vi "CoboltLaser_DriveCurrentGet.vi"(0 "ComPort":refnum<visa-resource-name>, 3 "CheckResponse":bool=TRUE, 7 "ErrorIn":errorcluster) -> (20 "ComPortOut":refnum<visa-resource-name>, 21 "LaserCurrent":dbl format="%.3g", 27 "ErrorOut":errorcluster)   [LabVIEW 2019]
doc: "Use this template to build a VI to use as a subVI."
panel:
  out "ResponseOK":bool
  out "Response":string
  # "(mA)"
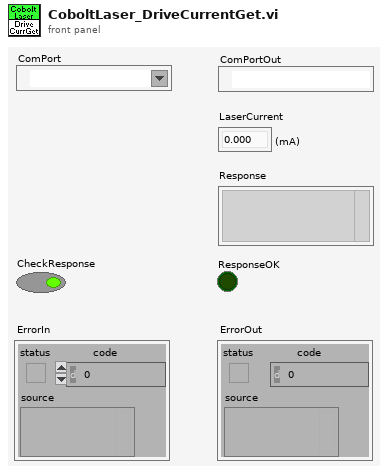
[diagram p1: front panel]
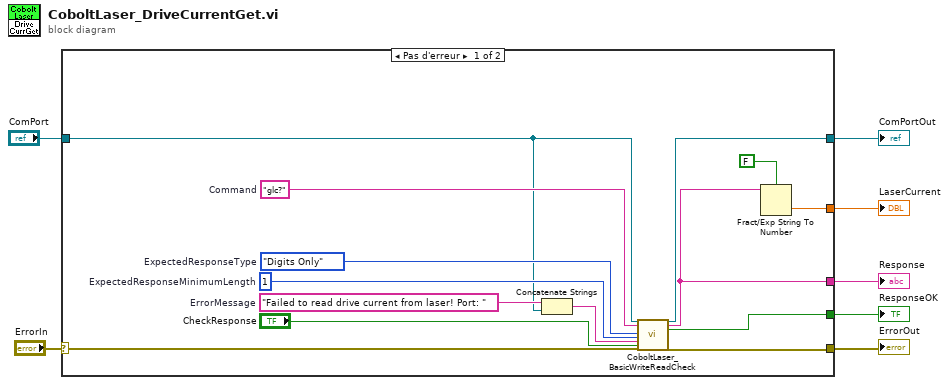
[diagram p0: block diagram]
diagram:
  n1 = case shown="Pas d'erreur" "ErrorIn" {
    selector: "ErrorIn" -> [w21 w23]
    tunnel: [w20 w23] -> w6
    tunnel: "ComPort" -> [w13 w22]
    tunnel: [w12 w22] -> w4
    tunnel: [w10 _] -> w3
    tunnel: [w9 _] -> w2
    tunnel: [w8 _] -> w1
    frame No Error {
      w17 = 1  # ExpectedResponseMinimumLength
      w18 = enum16{"Any", "Digits Only", "Non-Digits Only"}."Digits Only"  # ExpectedResponseType
      w15 = "Failed to read drive current from laser! Port: "  # ErrorMessage
      w19 = "glc?"  # Command
      n2 = Concatenate Strings(w15, w13) -> (w14:string)
      n3 = call <userlib>:"CoboltLaser_BasicWriteReadCheck.vi"("ComPort"=w13, "Command"=w19, "ExpectedResponseType"=w18, "ExpectedResponseMinimumLength"=w17, "ErrorMessage"=w14, "GenerateError"="CheckResponse", "error in (no error)"=w21) -> ("ComPortOut"=w12:refnum<visa-resource-name>, "Response"=w9:string, "ResponseOK"=w8:bool, "error out"=w20:errorcluster)  [unwired: 17 in]
      n4 = Fract/Exp String To Number(use system decimal point (T)=FALSE, string=w9) -> (number=w10:dbl)  [unwired: 2 in, 1 out]
    }
    frame Error {
    }
  }
  "ErrorOut" <- w6
  "ComPortOut" <- w4
  "Response" <- w2
  "ResponseOK" <- w1
  "LaserCurrent" <- w3
